vi "Get Channels per Device.vi"(8 "error in (no error)":errorcluster, 11 "RIO Target in":refnum<class "RIO Target.lvclass">) -> (0 "error out":errorcluster, 2 "Channels per Device":string[][](array[string]), 3 "RIO Target out":refnum<class "RIO Target.lvclass">)   [LabVIEW 2014, in "RIO Target.lvclass"]
uses:
  RIO Target.lvclass
  <vilib>/NI/Configuration Framework/Node/NISE_CEF_Node.lvclass/NISE_CEF_Node.ctl
  Bus/Bus.lvclass
  Device node/Device.lvclass
  Device Configuration/Device Configuration.lvclass
  Device Configuration/Device Configuration.lvclass/Device Configuration.ctl
  <vilib>/NI/Configuration Framework/Node/NISE_CEF_Node.lvclass
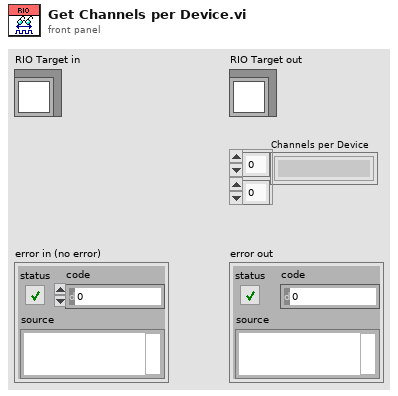
[diagram p1: front panel]
types:
  T1 = typedef "NISE_CEF_Node.lvclass/NodeRef.ctl" = refnum<data-value>
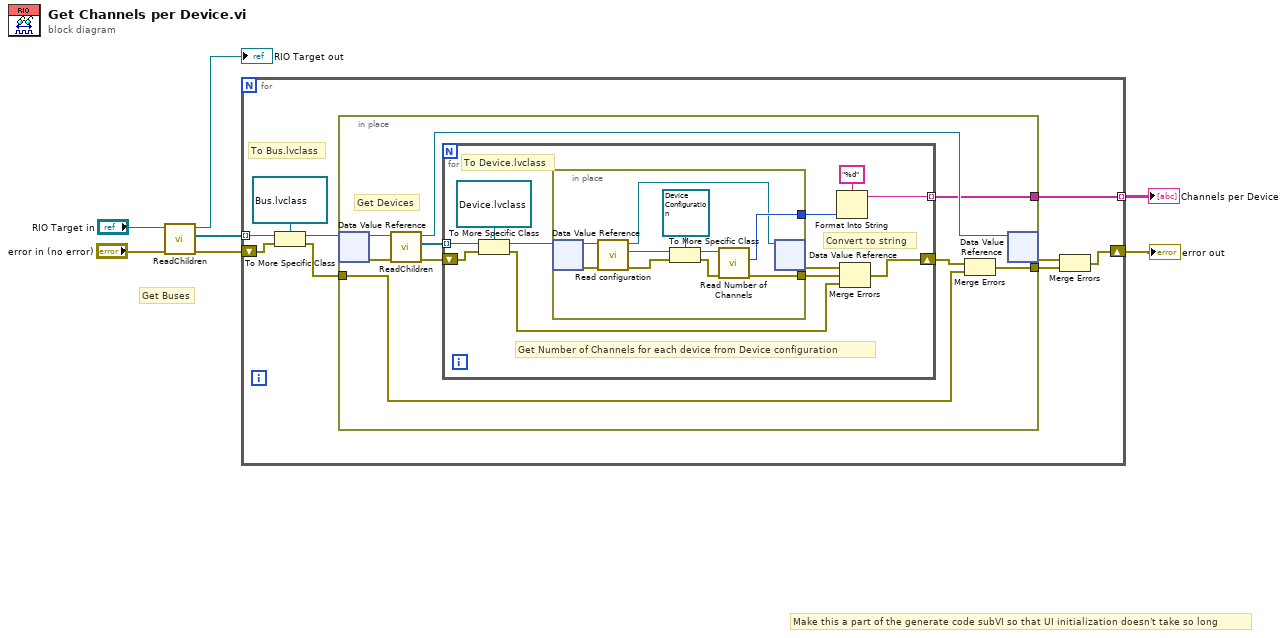
[diagram p0: block diagram]
diagram:
  # "Get Buses"
  # "Make this a part of the generate code subVI so that UI initialization doesn't take so long"
  n1 = call <vilib>:"ReadChildren.vi"("error in"="error in (no error)", "node in"="RIO Target in") -> ("error out"=w1:errorcluster, "output array"=w3:T1[], "node out"=→"RIO Target out":refnum<class "RIO Target.lvclass">)  [unwired: 7 in]
  n2 = for {
    tunnel: w3 -> [w16] mode=indexing
    tunnel: [w13] -> w7 mode=indexing
    shift-right: [w8] -> w6
    shift-left: w1 -> [w12]
    # "To Bus.lvclass"
    n3 = To More Specific Class(target class=refnum<data-value> refnum ("data value reference"), reference=w16, error in=w12) -> (specific class reference=w14:refnum<data-value>, error out=w11:errorcluster)
    n4 = in-place {
      in-place-border: [w23] -> w13
      in-place-border: w11 -> [w18]
      in-place-border: [w17] -> w9
      # "Get Devices"
      n5 = in-place-dvr #1(w14) -> (w22:refnum<class "Bus.lvclass">, w21:errorcluster)
      n6 = call <vilib>:"ReadChildren.vi"("error in"=w21, "node in"=w22) -> ("error out"=w20:errorcluster, "output array"=w25:T1[], "node out"=w24:refnum<class "Bus.lvclass">)  [unwired: 7 in]
      n7 = for {
        tunnel: w25 -> [w36] mode=indexing
        tunnel: [w33] -> w23 mode=indexing
        shift-right: [w27] -> w19
        shift-left: w20 -> [w30]
        # "Convert to string"
        # "Get Number of Channels for each device from Device configuration"
        # "To Device.lvclass"
        n8 = To More Specific Class(target class=refnum<data-value> refnum ("data value reference"), reference=w36, error in=w30) -> (specific class reference=w34:refnum<data-value>, error out=w26:errorcluster)
        n9 = in-place {
          in-place-border: [w39] -> w31
          in-place-border: [w37] -> w28
          n10 = in-place-dvr #2(w34) -> (w46:refnum<class "Device.lvclass">, w42:errorcluster)
          n11 = call-dynamic "Read configuration.vi"("error in"=w42, "Device in"=w46) -> ("error out"=w41:errorcluster, "configuration"=w45:refnum<class "NISE_CEF_serializable configuration.lvclass">, "Device out"=w38:refnum<class "Device.lvclass">)  [unwired: 7 in]
          n12 = To More Specific Class(target class=refnum<class "Device Configuration.lvclass"> refnum ("Device Configuration.lvclass"), reference=w45, error in=w41) -> (specific class reference=w43:refnum<class "Device Configuration.lvclass">, error out=w40:errorcluster)
          n13 = call "Read Number of Channels.vi"("error in (no error)"=w40, "Device Configuration in"=w43) -> ("error out"=w37:errorcluster, "Number of Channels"=w39:u32)  [unwired: 7 in, 1 out]
          n14 = in-place-dvr #2(w38) -> (w29:errorcluster)  [unwired: 1 out]
        }
        n15 = Format Into String(format string="%d", w31) -> (resulting string=w33:string)  [unwired: 2 in, 1 out]
        n16 = Merge Errors(w29, w28, w26) -> (w27:errorcluster)
      }
      n17 = Merge Errors(w19, w18) -> (w17:errorcluster)
      n18 = in-place-dvr #1(w24) -> (w10:errorcluster)  [unwired: 1 out]
    }
    n19 = Merge Errors(w10, w9) -> (w8:errorcluster)
  }
  "Channels per Device" <- w7
  "error out" <- w6
